vi "setHeaveConf.vi"(8 "error in (no error)":errorcluster, 11 "pHandle":u32) -> (0 "error out":errorcluster, 2 "return type":i32)   [LabVIEW 2011, in "sbgLabView.lvlib"]
uses:
  sbgLabView.lvlib
  sbgMatLab.dll
panel:
  in  "enableHeave":bool
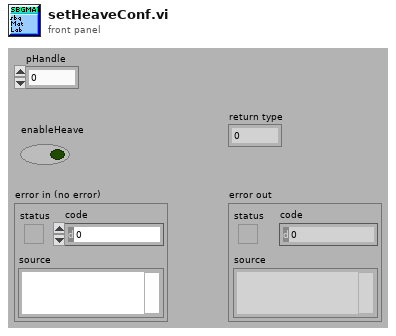
[diagram p1: front panel]
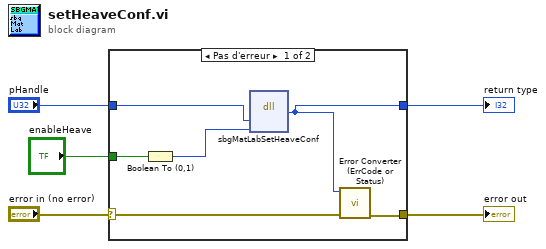
[diagram p0: block diagram]
diagram:
  n1 = case shown="Pas d'erreur" "error in (no error)" {
    selector: "error in (no error)" -> [w9 w12]
    tunnel: [w8 w12] -> w4
    tunnel: [w11 _] -> w3
    tunnel: "pHandle" -> [w10 _]
    tunnel: "enableHeave" -> [w7 _]
    frame No Error {
      n2 = Boolean To (0,1)(Boolean=w7) -> (0, 1=w6:i16)
      n3 = dll-call lib="C:/SBG-Systems/remote/projects/software/projects/labviewExample/sbgLabView/sbgMatLab.*" fn="sbgMatLabSetHeaveConf" ("sbgMatLab.dll:sbgMatLabGetMagneticDeclination")("pHandle"=w10, "enableHeave"=w6) -> ("type de retour"=w11:i32)  [unwired: 5 in, 2 out]
      n4 = call "Error Converter (ErrCode or Status).vi"("error in (no error)"=w9, "error code"=w11) -> ("error out"=w8:errorcluster)  [unwired: 9 in]
    }
    frame Error {
    }
  }
  "return type" <- w3
  "error out" <- w4
